vi "Create cursors.vi"(0 "Display State In":T1, 5 "Cursor pairs":u32, 9 "Container State":T2, 11 "error in (no error)":errorcluster) -> (4 "Display State Out":T1, 15 "error out":errorcluster)   [LabVIEW 2014, in "Graph with cursors XControl.xctl"]
uses:
  Graph with cursors XControl.xctl
  <vilib>/_xctls/Container State.ctl
  Graph with cursors State.ctl
  <vilib>/_xctls/XControlSupport.lvlib
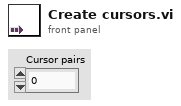
[diagram p1: front panel]
types:
  T1 = typedef "Graph with cursors XControl.xctl/Graph with cursors State.ctl" = cluster{"Cursor names":string[], "Cursor positions":dbl[], "Cursor pairs":i32, "Graph":refnum<vi>, "Prefix":string, "Base path":path}
  T2 = typedef "XControlSupport.lvlib/Container State.ctl" = cluster{"Indicator?":bool, "Run Mode?":bool, " Refnum":refnum<vi>}
  T3 = cluster{"Name":string, "Color":u32, "Style":u8, "Point Style":u8, "Name Visible":bool, "Allow Drag":bool, "Cursor Mode":u32, "Plot":i32, "Index":i32, "Position":cluster{"X":dbl, "Y":dbl}, "X Scale":u32, "Y Scale":u32, "Watch Plots":i32[], "Watch All Plots":bool, "Plot Area":i32, "Label Offset":cluster{"X":dbl, "Y":dbl}}[]
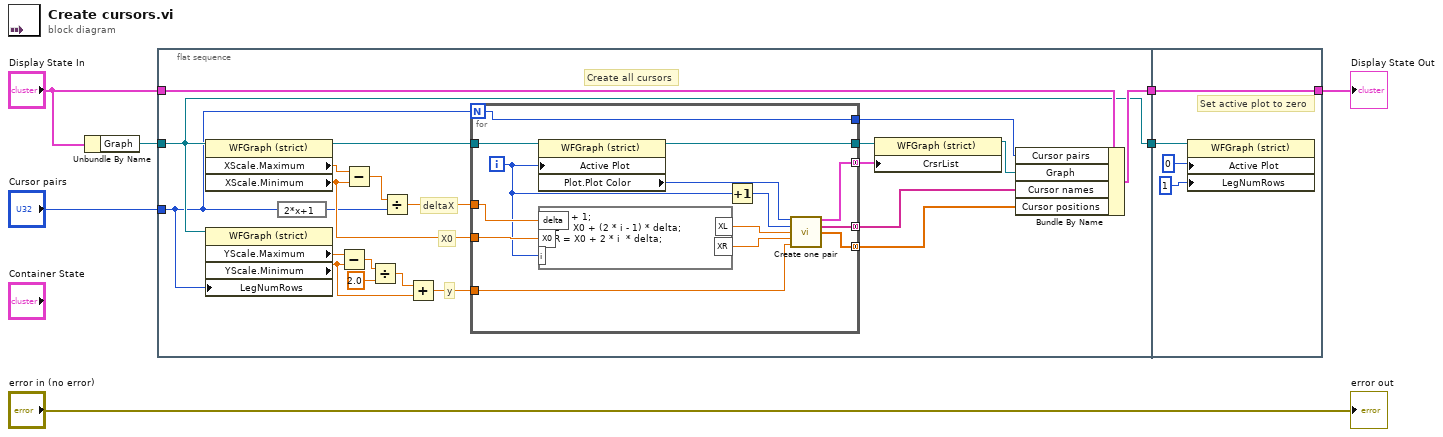
[diagram p0: block diagram]
diagram:
  n1 = Unbundle By Name("Display State In") -> ("Graph"=w5:refnum<vi>)
  n2 = flat-sequence {
    tunnel: [w9] -> w2
    tunnel: [w10] -> w1
    tunnel: "Cursor pairs" -> [w8]
    tunnel: w5 -> [w9]
    tunnel: "Display State In" -> [w11]
    tunnel: w2 -> [w46]
    tunnel: [w44] -> w3
    tunnel: w1 -> [w44]
    frame #0 {
      # "Create all cursors"
      # "X0"
      # "deltaX"
      # "y"
      n3 = property on="Property Node" class="WFGraph (strict)"(reference=w9) -> (reference out=w18:refnum<vi>, "XScale.Maximum"=w28:dbl, "XScale.Minimum"=w29:dbl)  [unwired: 1 in, 1 out]
      n4 = property on="Property Node" class="WFGraph (strict)"(reference=w9, "LegNumRows"=w8) -> ("YScale.Maximum"=w22:dbl, "YScale.Minimum"=w19:dbl)  [unwired: 1 in, 2 out]
      n5 = expression code="2*x+1"(w8) -> (w23:u32)
      n6 = Subtract(x=w22, y=w19) -> (x-y=w21:dbl)
      n7 = Subtract(x=w28, y=w29) -> (x-y=w27:dbl)
      n8 = Divide(x=w21, y=2.0) -> (x/y=w20:dbl)
      n9 = Divide(x=w27, y=w23) -> (x/y=w26:dbl)
      n10 = Add(x=w20, y=w19) -> (x+y=w24:dbl)
      n11 = for {
        N: w8 -> [w32]
        tunnel: w26 -> [w41]
        tunnel: w24 -> [w37]
        tunnel: w29 -> [w40]
        tunnel: w18 -> [w38]
        tunnel: [w36] -> w16 mode=concatenating
        tunnel: [w35] -> w14 mode=concatenating
        tunnel: [w34] -> w13 mode=concatenating
        tunnel: [w33] -> w17
        tunnel: [w32] -> w12
        i -> [w30]
        n12 = property on="Property Node" class="WFGraph (strict)"(reference=w38, "Active Plot"=w30) -> (reference out=w33:refnum<vi>, "Plot.Plot Color"=w39:u32)  [unwired: 1 in, 1 out]
        n13 = formula code="i = i + 1;\nXL = X0 + (2 * i - 1) * delta;\nXR = X0 + 2 * i  * delta;"("X0"=w40, "i"=w30, "delta"=w41) -> ("XL"=w43:dbl, "XR"=w42:dbl)
        n14 = Increment(x=w30) -> (x+1=w31:i32)
        n15 = call "Create one pair.vi"("Color"=w39, "Number"=w31, "XL"=w43, "XR"=w42, "Y"=w37) -> ("Cursors"=w36:T3, "Names"=w35:string[], "Xs"=w34:dbl[])  [unwired: 8 in]
      }
      n16 = property on="Property Node" class="WFGraph (strict)"(reference=w17, "CrsrList"=w16) -> (reference out=w15:refnum<vi>)  [unwired: 1 in, 1 out]
      n17 = Bundle By Name(cluster=w11, "Cursor pairs"=w12, "Graph"=w15, "Cursor names"=w14, "Cursor positions"=w13) -> (w10:T1)
    }
    frame #1 {
      # "Set active plot to zero"
      n18 = property on="Property Node" class="WFGraph (strict)"(reference=w46, "Active Plot"=u32 0 ("Legend:Number of Rows"), "LegNumRows"=u32 1 ("Legend:Number of Rows")) -> ()  [unwired: 1 in, 2 out]
    }
  }
  "Display State Out" <- w3
  "error out" <- "error in (no error)"
